vi "LHF.DB.Mongo.Util.VariantToUpdate.vi"(0 "Set":variant, 5 "error in (no error)":errorcluster) -> (14 ".NET Refnum out":refnum<k24>, 19 "error out":errorcluster)   [LabVIEW 2013, in "LHF.DB.Mongo.lvclass"]
uses:
  LHF.DB.Mongo.lvclass
  C:/Users/Ricardo/Desktop/Projetos/LabVIEW-MongoDB/src/Driver/MongoDB.Driver.dll
  Driver/MongoDB.Driver.dll
  <vilib>/Utility/VariantDataType/VariantType.lvlib
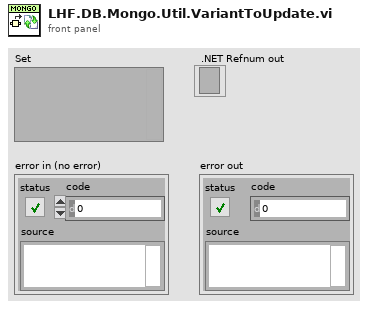
[diagram p1: front panel]
types:
  T1 = typedef "VariantType.lvlib/Type.ctl" = enum8{"Invalid Type", "Void", "I8", "I16", "I32", "I64", "U8", "U16", "U32", "U64", "Single Float", "Double Float", "Extended Float", "Single Complex", "Double Complex", "Extended Complex", "Enum U8", "Enum U16", "Enum U32", "Enum U64", "Single Float With Unit", "Double Float With Unit", "Extended Float With Unit", "Single Complex with Unit", "Double Complex with Unit", "Extended Complex with Unit", "Boolean", "String", "Path", "Picture", "Tag", "Array", "Cluster", "Variant", "LV Variant", "Waveform", "Timestamp", "Digital Waveform", "Digital Data", "ExpressData", "Refnum", "External Data", "VI", "Poly VI", "LabVIEW Class Instance", "Fixed Point"}
  T2 = typedef "LHF.DB.Mongo.lvclass/LHF.DB.Mongo.Typedef.VariantData.ctl" = cluster{"Type Enum":T1, "Name":string, "Variant":variant}
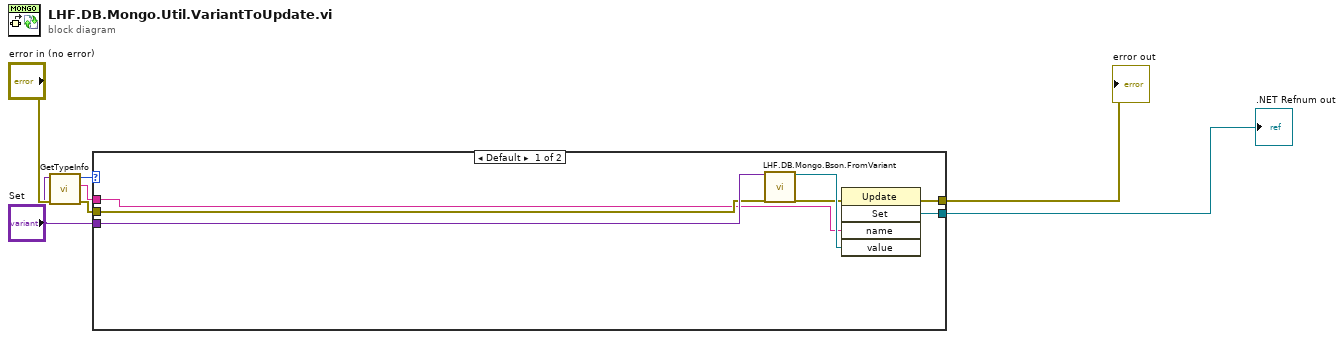
[diagram p0: block diagram]
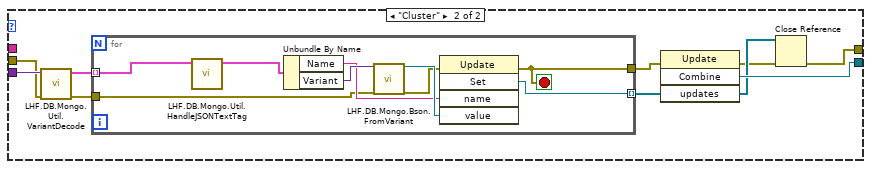
[diagram p2: hidden frame]
diagram:
  n1 = call <vilib>:"GetTypeInfo.vi"("error in (no error)"="error in (no error)", "Variant"="Set") -> ("error out"=w6:errorcluster, "Name"=w7:string, "Type Enum"=w1:T1)  [unwired: 5 in, 2 out]
  n2 = case shown="Default" w1 {
    tunnel: "Set" -> [w14 w24]
    tunnel: [w12 w21] -> w3
    tunnel: [w11 w16] -> w4
    tunnel: w6 -> [w10 w15]
    tunnel: w7 -> [w9 _]
    frame Default {
      n3 = call "LHF.DB.Mongo.Bson.FromVariant.vi"("Variant"=w14, "error IO"=w10) -> ("BsonValue"=w13:refnum<k24>, "error IO 2"=w8:errorcluster)  [unwired: 16 in]
      n4 = invoke class="Update" method="Set"(error in=w8, "name"=w9, "value"=w13) -> (error out=w11:errorcluster, "Set"=w12:refnum<k24>)  [unwired: 2 in, 3 out]
    }
    frame "Cluster" {
      n5 = call "LHF.DB.Mongo.Util.VariantDecode.vi"("error in (no error)"=w15, "variant"=w24) -> ("error out"=w20:errorcluster, "Variant Data"=w23:T2[])  [unwired: 7 in, 1 out]
      n6 = for {
        tunnel: w23 -> [w33] mode=indexing
        tunnel: [w28] -> w22 mode=indexing
        tunnel: w20 -> [w27]
        tunnel: [w25] -> w19
        stop <- w25 stop-if-true
        n7 = call "LHF.DB.Mongo.Util.HandleJSONTextTag.vi"("Variant Data"=w33) -> ("Variant Data (tag stripped)"=w32:T2)  [unwired: 9 in, 1 out]
        n8 = Unbundle By Name(w32) -> ("Name"=w29:string, "Variant"=w31:variant)
        n9 = call "LHF.DB.Mongo.Bson.FromVariant.vi"("Variant"=w31, "error IO"=w27) -> ("BsonValue"=w30:refnum<k24>, "error IO 2"=w26:errorcluster)  [unwired: 16 in]
        n10 = invoke class="Update" method="Set"(error in=w26, "name"=w29, "value"=w30) -> (error out=w25:errorcluster, "Set"=w28:refnum<k24>)  [unwired: 2 in, 3 out]
      }
      n11 = invoke class="Update" method="Combine"(error in=w19, "updates"=w22) -> (error out=w17:errorcluster, "Combine"=w21:refnum<k24>, "updates"=w18:refnum<k24>[])  [unwired: 2 in, 1 out]
      n12 = Close Reference(reference=w18, error in (no error)=w17) -> (error out=w16:errorcluster)
    }
  }
  "error out" <- w4
  ".NET Refnum out" <- w3
